vi "Parse Common Prefixes.vi"(8 "error in (no error)":errorcluster, 11 "Response body":string) -> (0 "error out":errorcluster, 3 "Common Prefixes":T1[](array[typedef]))   [LabVIEW 2015, in "NI_AWS_S3.lvlib" / "Object.lvlib"]
doc: "Parse out the CommonPrefixes part of the Response body of a List bucket request."
uses:
  Object.lvlib
  Common Prefix.ctl
  NI_AWS_S3.lvlib
  XML Parsing/NI_XML Parsing.lvlib
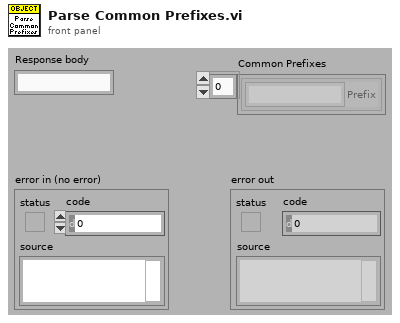
[diagram p1: front panel]
types:
  T1 = typedef "NI_AWS_S3.lvlib/Common Prefix.ctl" = cluster{"Prefix":string}
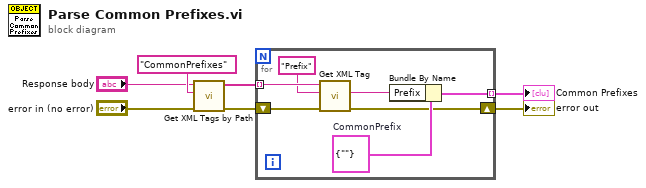
[diagram p0: block diagram]
diagram:
  n1 = call "Get XML Tags by Path.vi"("error in (no error)"="error in (no error)", "Tag path"="CommonPrefixes", "XML String in"="Response body") -> ("error out"=w5:errorcluster, "Matching tag values"=w6:string[])  [unwired: 7 in]
  n2 = for {
    tunnel: w6 -> [w13] mode=indexing
    shift-right: [w8] -> w2
    shift-left: w5 -> [w14]
    tunnel: [w9] -> w1 mode=indexing
    w11 = T1 {"Prefix"=""}  # CommonPrefix
    n3 = call "Get XML Tag.vi"("error in (no error)"=w14, "Tag name"="Prefix" ("Tag path"), "XML String in"=w13) -> ("error out"=w8:errorcluster, "Tag value"=w10:string)  [unwired: 4 in, 3 out]
    n4 = Bundle By Name(cluster=w11, "Prefix"=w10) -> (w9:T1)
  }
  "Common Prefixes" <- w1
  "error out" <- w2
